vi "GetSetFrameworkData.vi"(7 "Set (F)":bool, 11 "clFrameworkData In":T1={"EvtINIFilePaths"=[], "BusClassInstances"=[], "PmuImpairINIFilePaths"=[], "FlagImpairINIFilePaths"=[], "NetImpairINIFilePaths"=[], "OutputToFileINIFilePaths"=[], "AppINIFilePaths"=[], "AppModuleID"=-1, "OutputToFileID"=-1}) -> (3 "clFrameworkData Out":T1={"EvtINIFilePaths"=[], "BusClassInstances"=[], "PmuImpairINIFilePaths"=[], "FlagImpairINIFilePaths"=[], "NetImpairINIFilePaths"=[], "OutputToFileINIFilePaths"=[], "AppINIFilePaths"=[], "AppModuleID"=-1, "OutputToFileID"=-1})   [LabVIEW 2014, in "Framework.lvlib"]
uses:
  Framework.lvlib
  TypeDefs/clFrameworkData.ctl
  Bus_class/Bus.lvclass
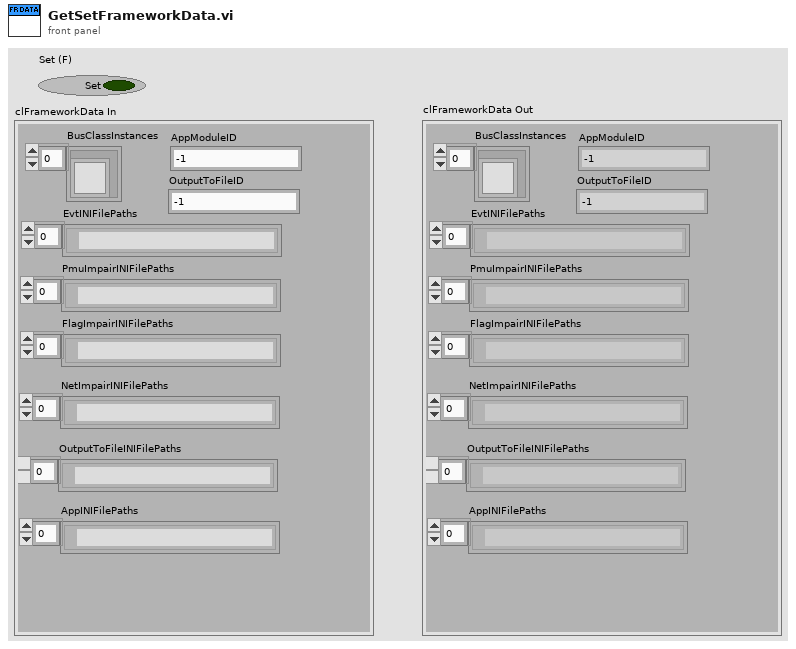
[diagram p1: front panel]
types:
  T1 = typedef "Framework.lvlib/clFrameworkData.ctl" = cluster{"EvtINIFilePaths":path[], "BusClassInstances":refnum<class "Bus.lvclass">[], "PmuImpairINIFilePaths":path[], "FlagImpairINIFilePaths":path[], "NetImpairINIFilePaths":path[], "OutputToFileINIFilePaths":path[], "AppINIFilePaths":path[], "AppModuleID":i32, "OutputToFileID":i32}
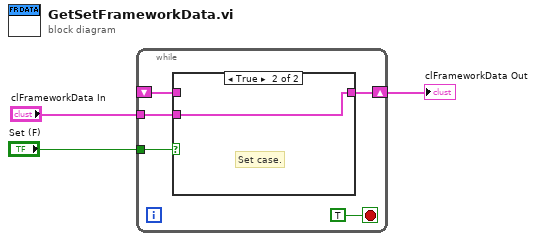
[diagram p0: block diagram]
diagram:
  n1 = while {
    tunnel: "Set (F)" -> [w7]
    shift-right: [w5] -> w2
    shift-left: _ -> [w6]
    tunnel: "clFrameworkData In" -> [w4]
    stop <- TRUE stop-if-true
    n2 = case shown="True" w7 {
      tunnel: w6 -> [w9 _]
      tunnel: [w9 w10] -> w5
      tunnel: w4 -> [_ w10]
      frame False {
        # "Get case."
      }
      frame True {
        # "Set case."
      }
    }
  }
  "clFrameworkData Out" <- w2
